vi "FdxCmdTxVLWriteExCvi.vi"(8 "error in":errorcluster, 9 "TxVLWriteInEx":T1 {"SequenceNumberControl" items=["FDX_TX_FRAME_SN_DEF", "FDX_TX_FRAME_SN_INC2", "FDX_TX_FRAME_SN_INC3", "FDX_TX_FRAME_SN_NO"]; "InterruptControl" items=["FDX_DIS", "FDX_ENA"]; "PreambleCount" items=["FDX_TX_FRAME_PRE_DEF", "1", "2 ", "3", "4", "5", "6", "7", "8", "9", "10", "11", "12", "13", "14", "n=15"]; "ExternalStrobe" items=["FDX_DIS", "FDX_ENA"]; "PhysErrorInjection" items=["FDX_TX_FRAME_ERR_OFF"=0, "FDX_TX_FRAME_ERR_CRC"=1, "FDX_TX_FRAME_ERR_ALI"=2, "FDX_TX_FRAME_ERR_PRE"=4, "FDX_TX_FRAME_ERR_PHY"=8]; "NetSelect" items=["FDX_TX_FRAME_DLY_A"=0, "FDX_TX_FRAME_DLY_B"=1, "FDX_TX_FRAME_BOTH "=3, "FDX_TX_FRAME_ONLY_A"=4, "FDX_TX_FRAME_ONLY_B "=5]}, 11 "InstrumentHandle":u32) -> (0 "error out":errorcluster, 1 "FramesWritten":u32, 3 "InstrumentHandle":u32)   [LabVIEW 2020, in "AIM664LV.lvlib"]
doc: "This function is used to write data directly to a virtual link buffer. The Virtual link has to be defined using function AiFdxCmdTxCreateVL."
uses:
  AIM664LV.lvlib
  AFDX_LibraryAdmin/FdxGlobalDllPath.vi
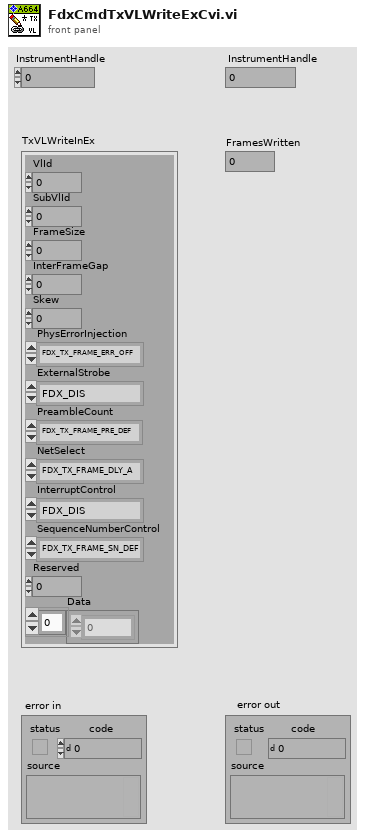
[diagram p1: front panel]
types:
  T1 = cluster{"VlId":u32, "SubVlId":u32, "FrameSize":u32, "InterFrameGap":u32, "Skew":u32, "Reserved":u32, "NetSelect":u32, "PhysErrorInjection":u32, "ExternalStrobe":u32, "PreambleCount":u32, "InterruptControl":u32, "SequenceNumberControl":u32, "Data":u8[]}
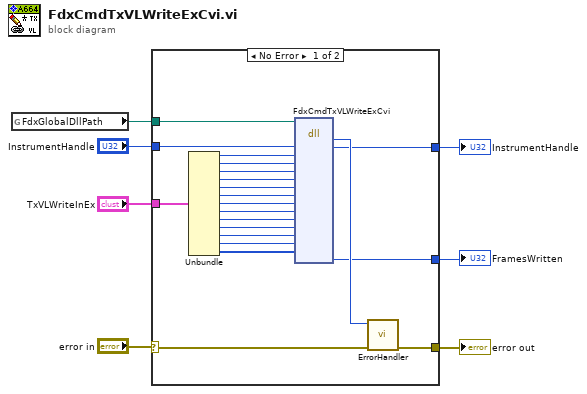
[diagram p0: block diagram]
diagram:
  n1 = global read "FdxGlobalDllPath.vi" "FdxGlobalDllPath"() -> (w5:path)
  n2 = case shown="No Error" "error in" {
    selector: "error in" -> [w27 w30]
    tunnel: [w28 w30] -> w7
    tunnel: w5 -> [w12 _]
    tunnel: "InstrumentHandle" -> [w11 w29]
    tunnel: [w10 w29] -> w3
    tunnel: "TxVLWriteInEx" -> [w9 _]
    tunnel: [w8 _] -> w1
    frame No Error {
      n3 = Unbundle(w9) -> ("VlId"=w25:u32, "SubVlId"=w24:u32, "FrameSize"=w23:u32, "InterFrameGap"=w22:u32, "Skew"=w21:u32, "Reserved"=w20:u32, "NetSelect"=w19:u32, "PhysErrorInjection"=w18:u32, "ExternalStrobe"=w17:u32, "PreambleCount"=w16:u32, "InterruptControl"=w15:u32, "SequenceNumberControl"=w14:u32, "Data"=w13:u8[])
      n4 = dll-call lib="aim_fdx.19.dll" fn="FdxCmdTxVLWriteExCvi"(path in=w12, "InstrumentHandle"=w11, "VlId"=w25, "SubVlId"=w24, "FrameSize"=w23, "InterFrameGap"=w22, "Skew"=w21, "PhysErrorInjection"=w20, "ExternalStrobe"=w19, "PreambleCount"=w18, "NetSelect"=w17, "InterruptControl"=w16, "SequenceNumberControl"=w15, "Reserved"=w14, "Data"=w13) -> ("status"=w26:i32, "InstrumentHandle"=w10:u32, "FramesWritten"=w8:u32)  [unwired: 15 in, 3 out]
      n5 = call "ErrorHandler.vi"("error in"=w27, "AIM Error"=w26) -> ("error out"=w28:errorcluster)  [unwired: 9 in]
    }
    frame Error {
    }
  }
  "error out" <- w7
  "InstrumentHandle" <- w3
  "FramesWritten" <- w1
